vi "2022_day04.vi"() -> ()   [LabVIEW 2021]
panel:
  out "Task 2":i32
  out "Task 1":i16
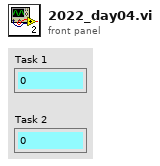
[diagram p1: front panel]
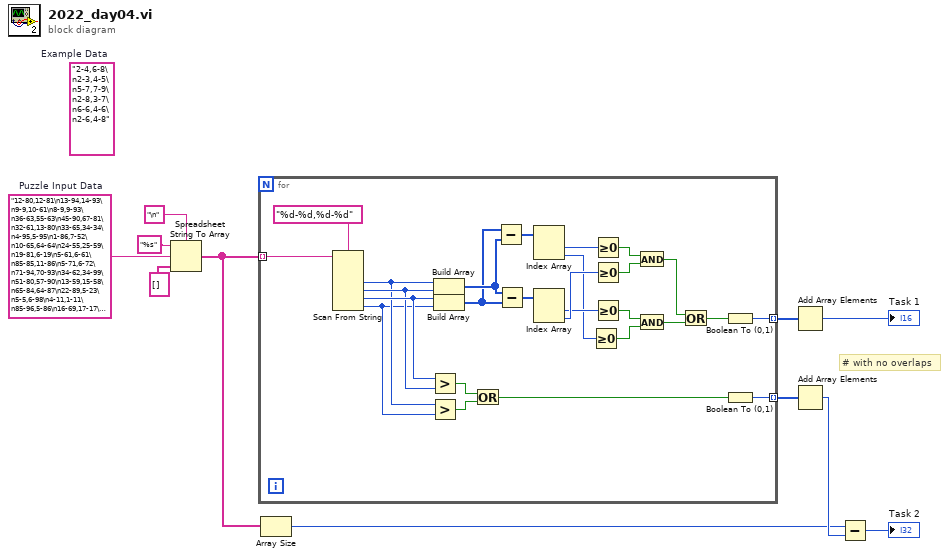
[diagram p0: block diagram]
diagram:
  w1 = "12-80,12-81\n13-94,14-93\n9-9,10-61\n8-9,9-93\n36-63,55-63\n45-90,67-81\n32-61,13-80\n33-65,34-34\n4-95,5-95\n1-86,7-52\n10-65,64-64\n24-55,25-59\n19-81,6-19\n5-61,6-61\n85-85,11-86\n5-71,6-72\n71-94,70-93\n34-62,34-99\n51-80,57-90\n13-59,15-58\n65-84,64-87\n22-89,5-23\n5-5,6-98\n4-11,1-11\n85-96,5-86\n16-69,17-17\n69-70,14-70\n35-98,35-58\n73-83,81-81\n13-93,92-92\n2-92,96-99\n10-10,10-99\n3-70,2-70\n81-89,3-81\n8-9,9-78\n6-99,75-98\n11-88,11-90\n31-92,32-93\n9-98,90-93\n29-87,27-29\n17-95,17-95\n29-86,85-87\n16-19,1-18\n22-93,19-62\n34-96,34-95\n89-91,47-90\n47-71,52-70\n11-29,10-28\n23-30,23-80\n5-92,5-87\n53-53,7-53\n61-73,22-73\n34-49,32-67\n54-82,53-55\n5-29,27-29\n15-77,14-66\n22-76,21-22\n87-88,15-88\n38-38,19-37\n2-98,2-97\n36-94,35-36\n2-45,3-45\n99-99,57-92\n36-96,38-97\n2-97,2-98\n11-98,11-99\n44-92,93-95\n8-94,8-74\n7-24,23-45\n16-40,16-41\n21-76,7-75\n2-5,4-20\n96-99,77-97\n1-20,9-23\n14-33,33-48\n26-35,26-34\n67-99,17-68\n22-22,21-90\n2-9,8-87\n64-74,6-65\n39-99,17-39\n14-55,21-80\n39-88,65-87\n19-98,19-97\n49-50,3-49\n3-71,3-72\n84-88,83-88\n22-35,22-36\n25-96,24-69\n12-36,3-20\n42-84,41-71\n4-99,4-47\n53-59,54-59\n21-95,20-96\n17-50,44-60\n25-81,26-82\n3-96,2-95\n13-40,12-71\n30-98,30-69\n55-60,54-61\n43-96,42-95\n12-35,28-35\n2-2,3-92\n7-82,3-6\n92-99,92-97\n44-63,44-73\n71-71,57-72\n93-93,8-94\n5-83,4-82\n18-42,41-41\n6-27,7-27\n64-82,15-81\n2-61,5-60\n14-50,51-51\n50-53,49-49\n22-88,22-89\n7-87,1-88\n14-14,9-15\n23-27,23-29\n14-91,14-92\n63-72,47-80\n32-32,31-98\n18-40,9-17\n19-23,18-21\n5-97,6-97\n35-93,18-94\n27-95,24-94\n14-22,21-45\n60-75,59-76\n6-90,6-90\n72-72,16-73\n24-28,85-92\n13-93,13-92\n25-94,24-95\n20-65,20-45\n2-6,7-88\n17-97,16-17\n3-37,3-98\n75-93,43-96\n99-99,10-87\n39-39,39-90\n26-56,25-63\n23-28,29-76\n40-86,39-40\n2-94,3-95\n76-76,75-77\n16-82,15-81\n14-14,13-99\n1-38,37-98\n7-32,8-21\n1-7,5-86\n3-69,3-3\n33-92,33-91\n81-85,82-86\n1-95,94-95\n2-83,2-3\n9-58,10-10\n42-50,42-49\n58-66,18-66\n14-33,13-33\n39-76,39-40\n9-96,8-35\n94-97,11-93\n1-82,2-74\n8-10,15-98\n25-49,15-50\n86-95,63-87\n61-79,71-78\n29-81,43-98\n58-60,16-59\n41-64,40-64\n51-98,51-51\n30-31,31-98\n61-94,45-61\n32-55,33-64\n80-81,37-81\n37-84,36-37\n40-40,41-91\n20-83,20-83\n16-23,17-22\n36-52,35-53\n21-86,24-90\n14-81,15-81\n18-76,18-98\n88-90,7-89\n98-99,8-94\n26-57,26-27\n98-98,2-97\n18-28,17-28\n34-63,56-89\n18-70,18-69\n66-88,40-87\n12-68,69-76\n55-77,78-87\n20-77,25-78\n73-86,4-99\n41-54,53-53\n25-60,59-60\n61-84,61-83\n27-43,26-42\n8-62,15-42\n3-63,15-62\n27-84,26-85\n24-87,2-25\n23-30,29-98\n10-61,9-60\n9-93,9-51\n90-91,7-91\n14-20,4-14\n96-99,27-97\n21-93,13-22\n23-74,73-73\n10-85,1-84\n34-75,72-72\n59-93,59-94\n87-93,49-96\n8-97,8-89\n98-98,14-96\n38-92,93-96\n35-36,36-95\n14-38,15-99\n55-91,73-91\n10-19,11-62\n17-93,4-56\n45-88,24-46\n75-78,28-71\n4-87,3-86\n67-94,67-93\n48-86,16-47\n12-58,8-57\n13-14,1-14\n66-69,33-79\n25-97,19-97\n38-55,28-39\n2-93,3-92\n28-65,30-64\n68-68,65-70\n29-85,30-86\n2-99,98-98\n7-64,33-98\n28-95,96-98\n72-82,72-81\n25-68,18-96\n81-84,82-86\n9-75,9-76\n96-99,42-94\n11-75,4-12\n20-89,47-88\n56-84,36-56\n24-73,24-84\n50-84,11-83\n29-99,2-93\n32-48,31-48\n49-49,48-86\n30-30,30-49\n56-97,36-96\n14-22,23-31\n90-90,3-90\n23-26,23-27\n31-49,31-50\n1-14,2-13\n10-73,10-72\n4-73,4-73\n26-92,91-94\n12-98,16-99\n50-91,38-39\n76-96,77-82\n17-98,51-96\n3-73,1-4\n1-99,98-99\n80-83,81-81\n24-58,25-25\n22-65,64-65\n1-2,3-95\n30-71,60-68\n46-46,17-45\n24-66,22-65\n4-97,6-97\n53-67,54-54\n16-90,20-89\n53-95,31-96\n17-44,18-29\n2-58,57-57\n63-63,3-63\n19-75,20-80\n13-60,13-60\n49-50,50-76\n32-48,33-48\n22-34,22-35\n7-29,18-86\n52-85,84-84\n90-99,72-94\n8-73,10-83\n50-50,36-51\n40-75,40-74\n67-93,67-76\n79-80,18-66\n92-95,6-91\n1-99,9-99\n24-32,24-31\n7-8,7-93\n5-99,21-81\n82-90,89-92\n58-58,3-57\n4-95,5-98\n85-88,84-87\n3-92,2-92\n48-90,48-89\n8-97,7-15\n26-62,61-61\n82-82,4-81\n19-32,21-32\n1-5,6-75\n37-37,36-63\n14-34,15-34\n26-46,10-47\n10-29,10-28\n58-86,1-60\n36-36,35-81\n25-60,26-59\n2-94,1-99\n5-39,8-39\n16-95,17-17\n4-96,4-96\n80-95,15-79\n41-41,24-41\n25-67,32-66\n10-37,11-38\n15-83,48-64\n2-6,5-36\n77-88,3-78\n35-95,35-96\n51-69,24-96\n71-96,45-97\n1-93,5-94\n19-92,93-93\n54-84,54-89\n7-86,18-87\n12-12,13-90\n90-95,16-91\n6-73,6-73\n9-27,8-23\n13-48,12-26\n9-55,54-54\n23-99,29-98\n56-74,73-74\n46-87,29-89\n97-97,47-98\n17-82,8-16\n2-84,2-97\n41-53,3-40\n6-16,6-64\n41-43,6-42\n2-41,3-40\n17-66,18-81\n2-2,1-99\n30-54,6-54\n70-81,69-69\n46-72,46-73\n18-87,17-86\n10-95,10-95\n28-79,23-89\n13-52,28-52\n2-24,2-24\n35-35,36-86\n35-74,35-85\n79-83,26-83\n4-60,4-88\n5-5,5-94\n6-35,34-87\n2-2,1-97\n59-94,93-95\n10-88,88-95\n48-88,45-89\n85-88,88-89\n16-39,15-80\n3-97,2-99\n26-56,27-59\n7-98,6-7\n64-84,64-98\n38-91,38-99\n43-97,43-98\n68-71,29-85\n32-89,38-89\n1-4,5-99\n6-86,6-38\n25-99,24-98\n2-99,59-97\n15-66,15-67\n53-74,53-73\n43-87,43-86\n9-73,7-73\n8-97,8-9\n69-73,70-71\n20-25,26-31\n20-26,25-99\n29-51,30-52\n18-28,19-35\n19-72,20-20\n27-80,2-60\n90-90,79-91\n30-67,66-68\n82-90,48-62\n9-11,10-90\n13-98,17-98\n8-13,7-12\n14-56,15-98\n25-97,24-24\n46-64,45-64\n80-89,80-81\n40-57,56-57\n49-50,32-50\n25-66,24-67\n21-68,21-26\n6-99,3-98\n11-63,11-90\n6-8,7-84\n9-75,8-74\n64-65,41-65\n17-17,17-34\n69-69,47-70\n2-10,10-64\n85-97,55-84\n72-72,40-71\n19-90,20-20\n5-84,83-85\n27-81,27-81\n21-98,28-61\n3-5,4-90\n25-67,23-25\n96-96,27-97\n11-11,10-97\n39-91,65-91\n29-60,59-60\n24-24,25-77\n72-73,72-98\n10-28,10-29\n8-97,36-85\n7-81,7-80\n39-50,38-39\n29-55,28-56\n7-98,6-97\n3-96,1-2\n43-99,42-98\n36-64,37-66\n26-96,96-96\n39-82,38-38\n10-98,11-99\n1-14,4-89\n3-63,1-99\n4-98,4-97\n79-80,2-80\n8-88,7-88\n47-58,44-57\n29-97,97-99\n21-63,20-22\n14-82,4-14\n20-72,45-71\n85-92,58-86\n15-29,15-30\n30-76,29-29\n19-50,13-51\n12-93,2-94\n14-20,21-87\n53-83,52-84\n2-14,2-84\n10-98,99-99\n2-98,3-99\n46-60,46-94\n8-69,63-70\n93-93,2-92\n40-81,49-80\n80-81,10-81\n17-67,5-68\n27-88,27-87\n92-92,14-91\n98-99,17-97\n7-53,1-7\n5-79,6-96\n2-18,4-65\n1-55,1-54\n46-60,59-59\n47-68,6-64\n4-26,5-22\n15-16,16-17\n51-52,49-52\n20-36,20-35\n1-29,1-98\n11-79,10-80\n25-69,43-79\n45-65,46-94\n35-35,24-38\n22-88,1-99\n14-65,15-65\n4-4,4-99\n1-87,82-87\n13-51,14-14\n9-82,3-10\n4-15,14-38\n26-86,48-53\n3-93,1-1\n22-22,23-48\n35-97,36-36\n1-94,1-95\n31-31,30-82\n3-30,3-75\n46-79,46-79\n43-73,13-87\n14-88,14-92\n41-95,42-95\n1-64,63-63\n3-98,97-98\n75-75,75-96\n11-52,12-51\n11-11,12-98\n30-92,55-93\n15-98,15-87\n25-40,22-95\n60-61,61-87\n6-19,18-90\n2-8,9-94\n61-90,42-60\n82-92,81-91\n1-33,1-48\n51-93,50-51\n47-74,48-75\n1-89,1-88\n65-67,28-66\n9-98,63-97\n91-92,12-92\n67-91,86-87\n48-89,86-89\n87-87,3-88\n8-79,78-78\n87-87,6-88\n46-46,46-75\n35-57,36-70\n9-51,9-12\n28-92,1-92\n52-65,24-66\n45-72,44-44\n42-48,41-46\n6-26,20-31\n10-48,48-49\n4-50,4-50\n23-75,75-83\n33-34,33-85\n49-70,49-70\n3-84,1-83\n20-92,21-91\n1-92,1-93\n2-81,1-96\n18-39,38-73\n61-82,60-81\n1-21,1-99\n28-31,30-31\n45-46,44-84\n57-95,58-94\n18-46,20-46\n43-87,14-90\n6-95,4-31\n15-61,16-73\n14-97,15-96\n15-86,16-16\n18-55,18-54\n24-99,24-97\n11-15,16-32\n12-12,12-93\n15-24,15-67\n7-62,30-58\n5-94,3-4\n87-99,3-53\n1-45,1-45\n31-68,30-31\n1-38,14-39\n43-96,42-43\n4-98,5-98\n76-90,7-91\n63-80,62-81\n6-98,15-97\n2-56,36-55\n9-32,10-33\n54-74,54-86\n71-80,2-84\n10-10,9-96\n24-44,25-43\n17-40,17-87\n7-56,1-55\n47-47,47-48\n25-66,25-65\n2-3,1-96\n65-65,65-66\n16-96,16-98\n87-92,11-93\n28-58,8-57\n2-60,59-60\n7-19,20-88\n30-54,31-55\n41-78,40-77\n45-61,44-44\n30-97,29-92\n10-37,2-46\n3-59,2-60\n9-69,9-88\n72-94,73-86\n37-42,41-41\n82-91,40-92\n40-97,24-40\n26-88,26-81\n43-61,4-62\n6-97,79-98\n38-61,60-60\n35-53,35-53\n64-64,63-73\n40-42,22-41\n28-57,50-56\n4-93,80-81\n2-50,2-59\n16-50,15-16\n11-74,75-75\n7-71,2-81\n9-94,9-95\n70-84,69-84\n2-99,3-99\n8-82,6-7\n9-93,9-98\n62-69,62-62\n26-91,30-92\n7-94,8-95\n73-73,1-74\n24-24,25-80\n3-96,1-1\n12-34,5-60\n2-96,97-99\n11-96,10-96\n12-90,7-93\n10-61,60-62\n36-51,50-52\n38-98,39-39\n9-97,9-81\n27-62,28-62\n28-71,29-29\n16-40,16-18\n51-95,33-71\n21-71,72-72\n58-66,66-66\n11-11,11-65\n26-86,26-88\n41-93,63-93\n37-47,37-46\n31-99,31-98\n75-90,75-95\n6-15,14-20\n6-85,6-37\n43-97,88-96\n95-95,96-96\n1-20,6-58\n23-45,29-44\n8-35,17-37\n44-71,45-71\n59-79,49-79\n39-73,40-74\n56-77,55-60\n45-45,45-71\n11-89,11-90\n43-52,51-51\n57-96,57-97\n89-91,89-90\n23-90,1-90\n2-98,2-9\n6-63,28-62\n29-29,28-98\n3-77,5-78\n39-69,38-74\n10-97,9-99\n6-19,6-20\n52-66,13-81\n30-30,29-70\n67-96,67-91\n72-91,71-83\n1-94,36-93\n8-9,9-98\n3-78,73-77\n31-97,31-96\n44-70,65-67\n42-66,50-67\n6-79,5-80\n30-36,21-37\n38-43,39-51\n51-51,52-81\n10-87,87-88\n19-27,18-19\n13-99,85-98\n59-89,88-88\n25-26,26-97\n31-74,75-75\n6-95,95-95\n30-71,70-72\n24-51,23-95\n55-77,56-76\n26-49,26-48\n34-56,34-57\n9-11,8-10\n1-98,1-97\n6-97,12-96\n35-72,35-75\n2-99,4-99\n4-92,3-93\n6-98,13-99\n2-85,84-86\n90-98,5-90\n59-84,60-85\n9-19,19-93\n15-71,19-65\n98-99,85-99\n8-25,24-26\n42-72,42-71\n52-81,81-82\n50-88,51-51\n87-87,9-86\n6-91,3-5\n10-83,3-82\n99-99,9-95\n68-69,68-68\n42-42,36-43\n28-58,27-58\n3-85,1-85\n8-88,8-89\n11-86,12-93\n21-60,1-99\n6-96,3-7\n73-91,83-85\n98-98,11-99\n31-69,28-70\n89-91,57-90\n5-95,10-94\n48-50,3-49\n12-76,10-13\n2-60,2-25\n2-33,34-72\n14-19,18-18\n34-86,35-87\n20-92,97-99\n11-83,83-84\n17-80,16-79\n96-99,4-97\n15-92,16-92\n24-99,81-97\n7-92,93-99\n24-80,25-90\n71-88,87-94\n6-64,32-69\n34-48,46-67\n13-14,14-63\n26-47,26-46\n18-33,18-33\n96-97,5-95\n49-93,48-94\n52-79,58-58\n2-62,3-63\n8-80,9-71\n41-75,32-40\n53-96,71-71\n85-85,84-84\n63-76,59-77\n58-76,59-75\n4-19,18-19\n1-98,3-99\n22-90,22-68\n9-96,97-97\n11-75,12-76\n9-45,9-46\n20-83,20-84\n8-83,5-84\n74-96,92-92\n3-95,4-95\n19-30,19-29\n71-81,8-71\n10-98,11-95\n3-90,4-90\n7-18,18-36\n9-21,4-21\n1-52,3-52\n21-61,21-61\n2-99,21-24\n31-92,58-97\n4-71,4-71\n16-40,17-64\n43-85,44-86\n4-62,61-62\n3-91,4-90\n64-64,35-63\n6-78,5-5\n59-71,33-72\n56-60,55-61\n3-76,1-77\n30-32,31-31\n23-78,25-69\n9-99,4-10\n19-85,9-88\n4-97,3-3\n75-96,74-96\n97-98,96-96\n10-97,10-98\n85-85,85-85\n4-49,4-48\n17-97,14-97\n4-4,3-89\n34-64,15-34\n19-83,19-19\n24-70,23-69\n18-40,17-62\n19-79,18-19\n30-82,30-58\n5-8,7-28\n2-8,4-85\n4-4,3-85\n10-41,11-40\n86-89,69-85\n44-71,71-84\n51-79,51-97\n20-97,64-97\n2-23,2-23\n8-29,22-28\n81-97,57-68\n69-84,68-84\n2-98,2-90\n23-42,29-56\n11-89,11-88\n14-72,10-79\n46-75,74-74\n52-54,48-53\n12-80,19-80\n4-62,3-62\n3-4,3-87\n1-2,4-84\n3-43,3-44\n56-94,94-94\n14-49,15-49\n54-58,55-58\n1-96,2-62\n32-70,17-70\n23-86,23-85\n5-97,2-96\n46-72,47-71\n90-90,25-90\n30-54,53-54\n4-88,34-45\n27-92,28-92\n38-39,38-85\n8-46,7-28\n5-66,5-67\n7-98,7-56\n39-85,39-86\n17-64,17-65\n50-88,49-88\n4-49,4-79\n14-72,14-71\n62-79,63-83\n2-75,2-21\n8-83,8-15\n72-94,77-77\n63-98,63-98\n52-56,52-70\n4-77,3-4\n73-81,73-73\n6-91,7-37\n33-86,2-80\n19-22,18-18\n2-98,4-77\n18-63,13-17\n29-40,30-41\n5-98,20-92\n24-78,20-23\n5-34,5-35\n97-99,15-98\n4-69,5-68\n74-76,63-76\n23-97,96-97\n7-94,7-93\n18-24,18-24\n28-45,45-45\n14-63,48-55\n10-69,10-68\n78-80,47-79\n33-72,32-32\n68-90,68-69\n52-58,59-72\n18-26,8-44\n11-96,6-97\n52-98,52-99\n64-96,63-82\n24-90,77-90\n2-73,82-85\n70-79,68-90\n8-74,13-75\n1-25,3-24\n1-94,6-52\n34-92,31-96\n36-78,35-79\n2-64,1-65\n41-90,20-91\n68-70,3-71\n51-53,51-59\n10-13,14-88\n33-95,33-94\n71-98,70-96\n1-93,4-88\n8-62,5-61\n39-90,40-91\n89-89,32-90\n1-11,1-10\n6-63,6-62\n22-85,11-51\n9-9,8-95\n9-79,9-73\n9-91,9-34\n62-85,20-61\n73-87,73-86\n15-45,17-45\n16-94,16-95\n1-18,4-57\n28-45,44-45\n14-62,13-61\n8-36,3-8\n12-50,44-49\n47-62,47-61\n16-78,15-64\n44-45,45-51\n3-25,6-26\n47-70,46-71\n28-83,13-84\n1-99,2-98\n19-76,19-77\n35-58,25-57\n4-63,1-3\n98-99,3-99\n28-89,89-90\n64-86,13-86\n66-89,42-67\n22-71,8-88\n91-94,1-92\n72-92,73-91\n13-28,13-65\n28-99,28-97\n59-81,59-80\n57-93,92-92\n71-98,71-81\n2-4,3-53\n20-65,30-65\n11-75,76-85\n1-90,1-89\n2-25,24-24\n64-91,63-93\n15-97,7-16\n33-64,42-63\n77-81,6-98\n7-91,8-92\n2-48,2-48\n63-65,32-64\n23-95,23-95\n41-41,52-94\n10-26,10-80\n99-99,2-57\n37-66,25-37\n17-81,18-81\n76-93,92-92\n58-89,9-59\n31-31,30-87\n46-85,84-86\n3-4,5-99\n37-95,37-40\n3-75,3-93\n44-86,42-44\n4-50,49-50\n20-43,19-43\n83-91,82-97\n39-39,38-77\n1-94,1-95\n53-74,30-54\n25-69,25-68\n3-85,85-85\n37-69,4-68\n57-84,53-57\n57-95,20-99\n9-85,9-84\n25-79,26-26\n5-99,3-98\n58-86,57-85\n3-24,4-59\n6-93,7-93\n74-96,75-96\n92-98,12-92\n55-62,49-56\n1-73,1-99\n8-99,98-99\n12-72,12-71\n52-72,71-71\n63-97,63-96\n21-99,20-21"  # Puzzle Input Data
  (unwired) "2-4,6-8\n2-3,4-5\n5-7,7-9\n2-8,3-7\n6-6,4-6\n2-6,4-8"  # Example Data
  # "# with no overlaps"
  n1 = Spreadsheet String To Array(delimiter (Tab)="\n", format string="%s", spreadsheet string=w1, array type (2D Dbl)=string[] []) -> (array=w5:string[])
  n2 = for {
    tunnel: w5 -> [w37] mode=indexing
    tunnel: [w34] -> w7 mode=indexing
    tunnel: [w13] -> w6 mode=indexing
    n3 = Scan From String(format string="%d-%d,%d-%d", input string=w37) -> (output 1=w17:i32, output 2=w18:i32, output 3=w19:i32, output 4=w16:i32)  [unwired: 6 in, 3 out]
    n4 = Greater?(x=w19, y=w18) -> (0:w14:bool)
    n5 = Greater?(x=w17, y=w16) -> (0:w15:bool)
    n6 = Build Array(w17, w18) -> (w33:i32[])
    n7 = Build Array(w19, w16) -> (w32:i32[])
    n8 = Or(x=w14, y=w15) -> (x .or. y?=w12:bool)
    n9 = Subtract(x=w32, y=w33) -> (x-y=w30:i32[])
    n10 = Subtract(x=w33, y=w32) -> (x-y=w31:i32[])
    n11 = Index Array(array=w30) -> (element #1=w28:i32, element #2=w24:i32)  [unwired: 2 in]
    n12 = Index Array(array=w31) -> (element #1=w25:i32, element #2=w27:i32)  [unwired: 2 in]
    n13 = Greater Or Equal To 0?(x=w24) -> (x >= 0?=w23:bool)
    n14 = Greater Or Equal To 0?(x=w28) -> (x >= 0?=w29:bool)
    n15 = Greater Or Equal To 0?(x=w27) -> (x >= 0?=w26:bool)
    n16 = Greater Or Equal To 0?(x=w25) -> (x >= 0?=w35:bool)
    n17 = And(x=w29, y=w26) -> (x .and. y?=w22:bool)
    n18 = And(x=w35, y=w23) -> (x .and. y?=w21:bool)
    n19 = Or(x=w22, y=w21) -> (x .or. y?=w20:bool)
    n20 = Boolean To (0,1)(Boolean=w20) -> (0, 1=w34:i16)
    n21 = Boolean To (0,1)(Boolean=w12) -> (0, 1=w13:i16)
  }
  n22 = Array Size(array=w5) -> (size(s)=w3:i32)
  n23 = Add Array Elements(numeric array=w7) -> (sum=→"Task 1":i16)
  n24 = Add Array Elements(numeric array=w6) -> (sum=w4:i16)
  n25 = Subtract(x=w3, y=w4) -> (x-y=→"Task 2":i32)
